vi "AI_Loop.vi"(8 "error in":errorcluster, 10 "AI_Type":T1=enum."TC") -> (0 "error out":errorcluster)   [LabVIEW 2018]
doc: "This example demonstrates how to continuously acquire buffered voltage measurements using a DAQmx device.\n\nFor instructions on how to connect your signals to the DAQ device, refer to your device documentation."
uses:
  Controls/Enums/AI_Type_Enum.ctl
  Controls/Enums/AI_Loop_Enum.ctl
  Controls/Clusts/AI_Loop_Clust.ctl
  Controls/Clusts/AllThresholds.ctl
  Controls/Clusts/ThresholdAlarmLimits.ctl
  Controls/Clusts/Inclinometer_User_Cfg.ctl
  Controls/Clusts/AlarmSettingsClust.ctl
  Controls/Clusts/AlarmThresh_OneChan.ctl
  Controls/Enums/LogLoopEnum.ctl
  Controls/Enums/FP_Loop_Enum.ctl
  Controls/Enums/WatchdogTimer_Enum.ctl
  <vilib>/DAQmx/read.llb/DAQmx Read (Analog 1D DBL NChan 1Samp).vi
  <vilib>/DAQmx/create/channels.llb/DAQmx Create Channel (AI-Voltage-Basic).vi
  <vilib>/DAQmx/create/channels.llb/DAQmx Create Channel (AI-Temperature-Thermocouple).vi
  <vilib>/DAQmx/miscellaneous.llb/DAQmx Fill In Error Info.vi
panel:
  out "Graph":dbl[](graph)
  # "Acquired Data"
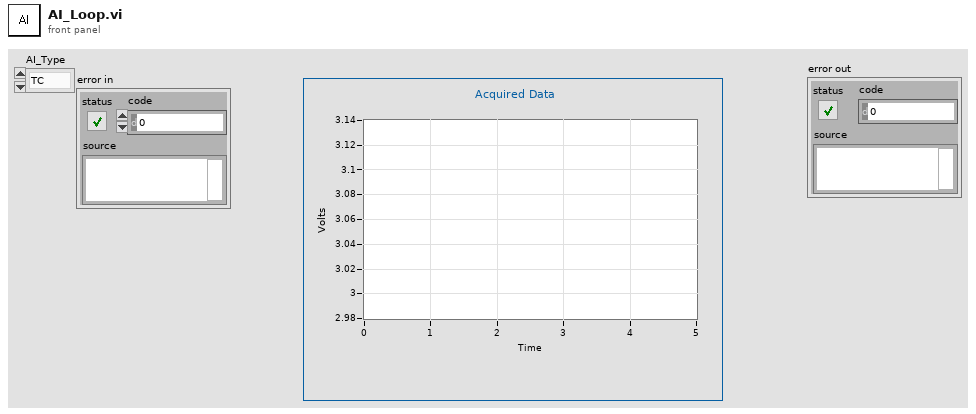
[diagram p1: front panel]
types:
  T1 = typedef "AI_Type_Enum.ctl" = enum16{"AI", "TC"}
  T2 = typedef "AI_Loop_Clust.ctl" = cluster{"AI_Type":T1, "task":refnum<k21>, "AllThresholds_deprecated":T3, "Inclin":T5, "Alarm":T6}
  T3 = typedef "AllThresholds.ctl" = cluster{"TC0":T4, "TC1":T4, "TC2":T4, "TC3":T4, "TC4":T4, "TC5":T4, "TC6":T4, "TC7":T4, "TC8":T4, "TC9":T4, "TC10":T4, "TC11":T4, "TC12":T4, "TC13":T4, "TC14":T4, "TC15":T4, "TC16":T4, "TC17":T4, "TC18":T4, "TC19":T4, "TC20":T4, "AI0":T4, "AI1":T4, "AI2":T4, "AI3":T4, "AI4":T4, "AI5":T4, "AI6":T4, "AI7":T4, "AI16":T4, "AI17":T4, "AI18":T4, "AI19":T4, "AI20":T4, "AI21":T4, "AI22":T4, "AI23":T4}
  T4 = typedef "ThresholdAlarmLimits.ctl" = cluster{"Enable":bool, "LoErr":dbl, "LoWarn":dbl, "HiWarn":dbl, "HiErr":dbl, "RX?":bool}
  T5 = typedef "Inclinometer_User_Cfg.ctl" = cluster{"Vmin":dbl, "Vmax":dbl, "Angle_min":dbl, "Angle_max":dbl, "Offset":dbl, "Pos_Neg":bool}
  T6 = typedef "AlarmSettingsClust.ctl" = cluster{"TC13":T7, "AI1":T7, "AI2":T7, "AI3":T7, "AI4":T7, "AI5":T7, "AI6":T7, "AI18":T7, "AI19":T7, "TE1":T7, "TE2":T7, "TE3":T7, "ADAM1":T7, "ADAM2":T7, "ADAM3":T7, "ADAM4":T7, "72CoBeacFreq":T7, "72CoCalFreq":T7, "84CoBeacFreq":T7, "84CoCalFreq":T7, "72Co_CalTonePwr":T7, "72X_CalTonePwr":T7, "84Co_CalTonePwr":T7, "84X_CalTonePwr":T7}
  T7 = typedef "AlarmThresh_OneChan.ctl" = cluster{"Enbl":bool, "ErrsAndWarns":cluster{dbl, dbl, dbl, dbl}}
  T8 = typedef "AI_Loop_Enum.ctl" = enum16{"AI_Init", "AI_Config", "AI_Alarm", "AI_Read", "AI_ChkTime", "AI_Exit"}
  T9 = typedef "WatchdogTimer_Enum.ctl" = enum16{"ResetAll", "CheckAll", "HW1", "HW2", "Tones", "FP", "Noise", "Log", "TCP", "AI", "TC", "ADAM", "Disdrom", "TE", "Weather"}
  T10 = typedef "FP_Loop_Enum.ctl" = enum16{"FP_Init", "FP_Scale", "FP_Tone", "FP_Noise", "FP_Probes", "FP_PXI", "FP_AI", "FP_TC", "FP_PWR_Hist", "FP_Alarm", "FP_Exit"}
  T11 = typedef "LogLoopEnum.ctl" = enum16{"Log_Init", "Log_Config", "Log_CfgAlarm", "Log_TimeDomain", "Log_Tone", "Log_NoiseTrace", "Log_NoiseSum", "Log_DO", "Log_AI", "Log_TC", "Log_Disdrom", "Log_Weather", "Log_TE", "Log_ADAM", "Log_UPS", "Log_ChkTime", "Log_Alarm", "Log_SSH", "Log_Write", "Log_Exit"}
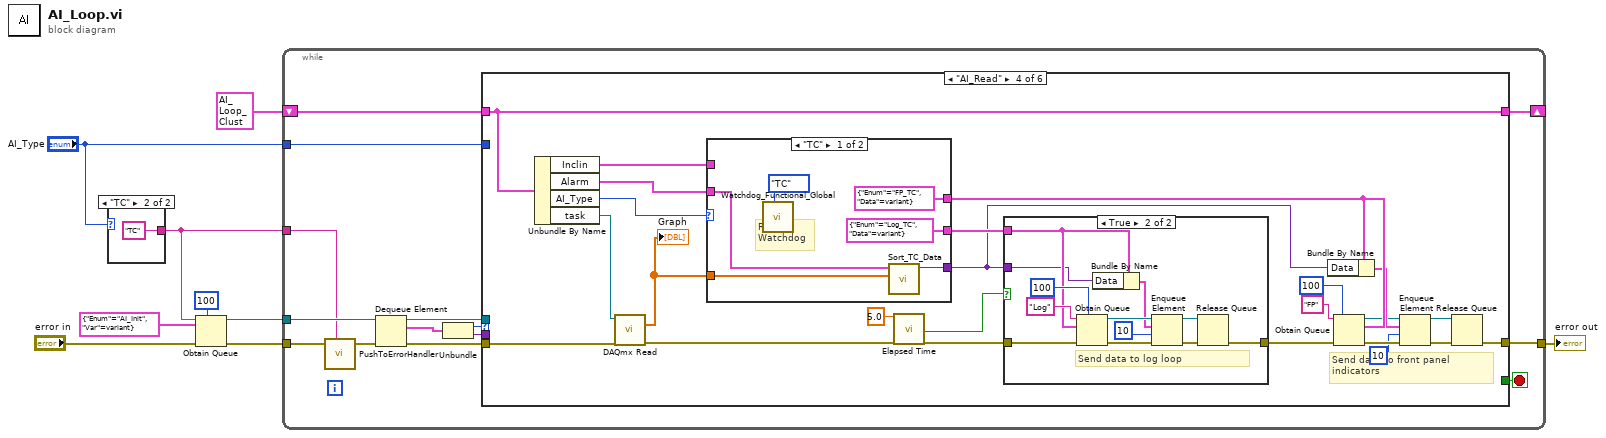
[diagram p0: block diagram]
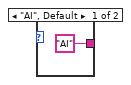
[diagram p2: hidden frame]
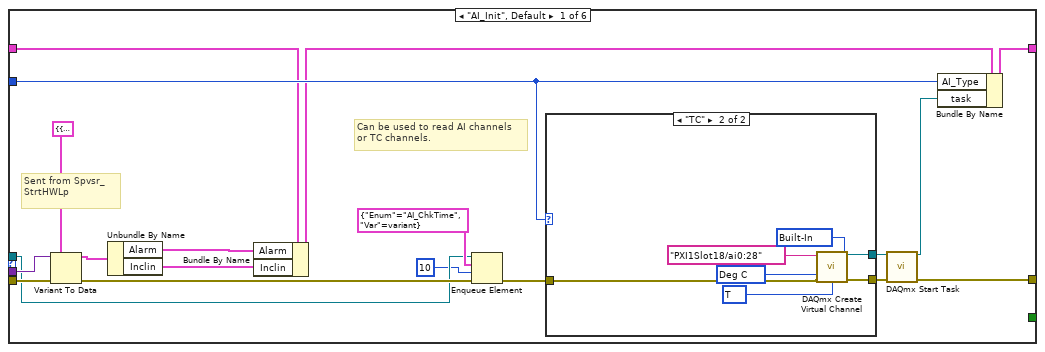
[diagram p3: hidden frame]
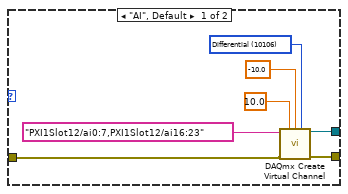
[diagram p4: hidden frame]
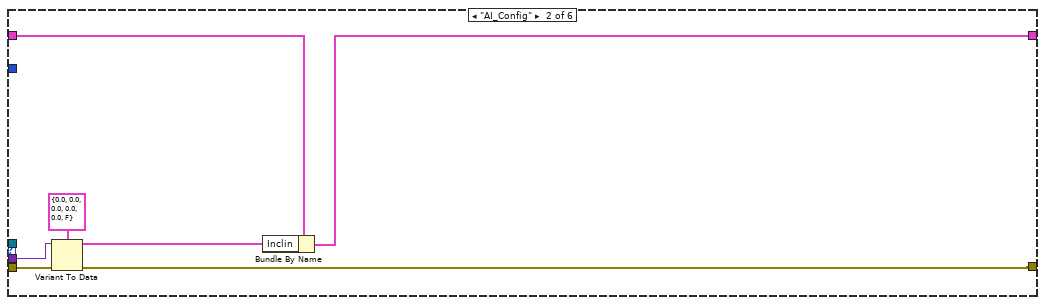
[diagram p5: hidden frame]
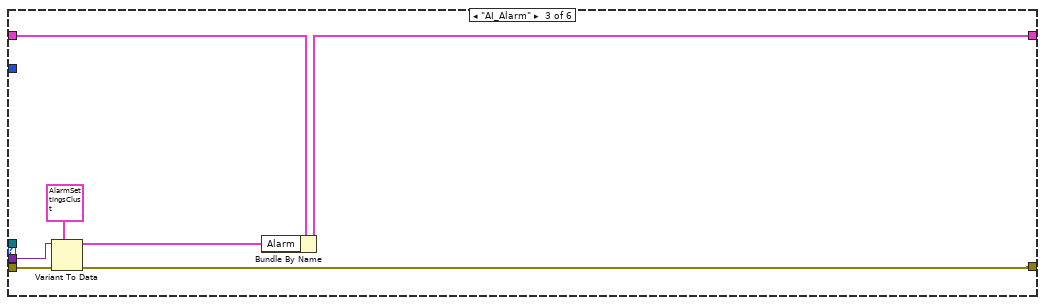
[diagram p6: hidden frame]
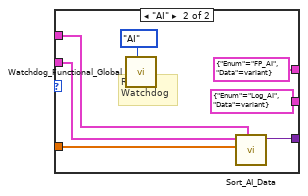
[diagram p8: hidden frame]
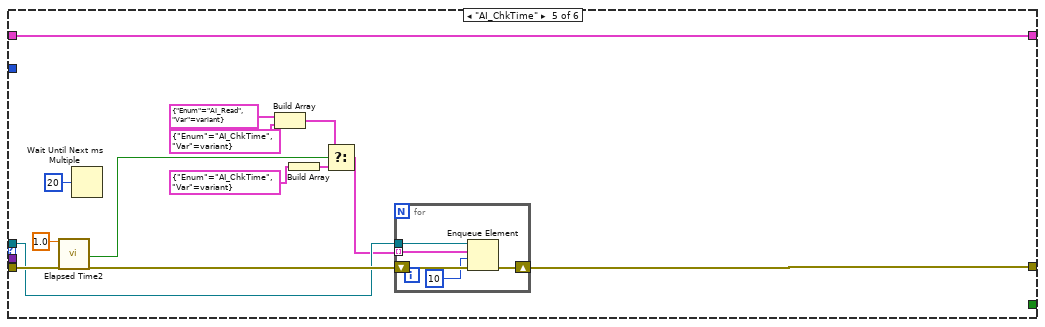
[diagram p9: hidden frame]
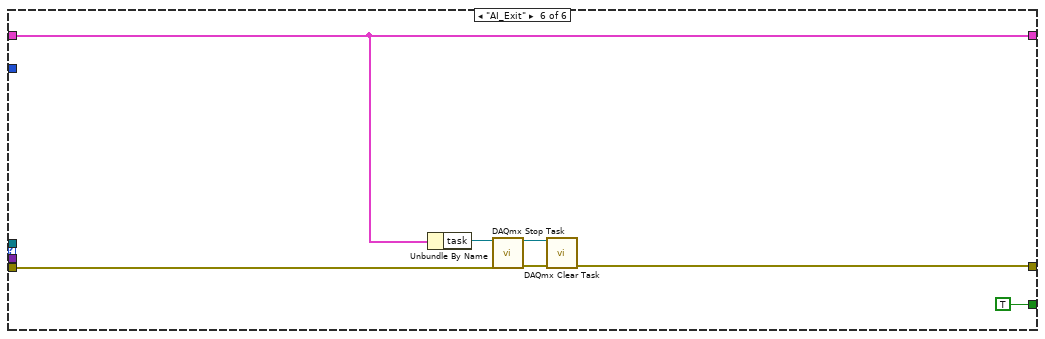
[diagram p10: hidden frame]
diagram:
  n1 = case shown="\"TC\"" "AI_Type" {
    tunnel: ["AI" ("name (unnamed)") "TC" ("name (unnamed)")] -> w4
    frame "AI", Default {
    }
    frame "TC" {
    }
  }
  n2 = Obtain Queue(max queue size (-1, unlimited)=100, name (unnamed)=w4, element data type=cluster{"Enum":T8, "Var":variant} {"Enum"=enum."AI_Init", "Var"=variant}, error in (no error)="error in") -> (queue out=w2:refnum<queue>, error out=w1:errorcluster)  [unwired: 1 in, 1 out]
  n3 = while {
    tunnel: w1 -> [w17]
    tunnel: [w25] -> w6
    tunnel: w2 -> [w19]
    tunnel: w4 -> [w14]
    shift-right: [w12] -> _
    shift-left: T2 {"AI_Type"=enum."TC", "task"="", "AllThresholds_deprecated"={"TC0"={"Enable"=FALSE, "LoErr"=34.0, "LoWarn"=60.0, "HiWarn"=90.0, "HiErr"=105.0, "RX?"=FALSE}, "TC1"={"Enable"=FALSE, "LoErr"=34.0, "LoWarn"=60.0, "HiWarn"=90.0, "HiErr"=105.0, "RX?"=FALSE}, "TC2"={"Enable"=FALSE, "LoErr"=34.0, "LoWarn"=60.0, "HiWarn"=90.0, "HiErr"=105.0, "RX?"=FALSE}, "TC3"={"Enable"=FALSE, "LoErr"=34.0, "LoWarn"=60.0, "HiWarn"=90.0, "HiErr"=105.0, "RX?"=FALSE}, "TC4"={"Enable"=FALSE, "LoErr"=34.0, "LoWarn"=60.0, "HiWarn"=90.0, "HiErr"=105.0, "RX?"=FALSE}, "TC5"={"Enable"=FALSE, "LoErr"=34.0, "LoWarn"=60.0, "HiWarn"=90.0, "HiErr"=105.0, "RX?"=FALSE}, "TC6"={"Enable"=FALSE, "LoErr"=34.0, "LoWarn"=60.0, "HiWarn"=90.0, "HiErr"=105.0, "RX?"=FALSE}, "TC7"={"Enable"=FALSE, "LoErr"=34.0, "LoWarn"=60.0, "HiWarn"=90.0, "HiErr"=105.0, "RX?"=FALSE}, "TC8"={"Enable"=FALSE, "LoErr"=34.0, "LoWarn"=60.0, "HiWarn"=90.0, "HiErr"=105.0, "RX?"=FALSE}, "TC9"={"Enable"=FALSE, "LoErr"=34.0, "LoWarn"=60.0, "HiWarn"=90.0, "HiErr"=105.0, "RX?"=FALSE}, "TC10"={"Enable"=FALSE, "LoErr"=34.0, "LoWarn"=60.0, "HiWarn"=90.0, "HiErr"=105.0, "RX?"=FALSE}, "TC11"={"Enable"=FALSE, "LoErr"=34.0, "LoWarn"=60.0, "HiWarn"=90.0, "HiErr"=105.0, "RX?"=FALSE}, "TC12"={"Enable"=FALSE, "LoErr"=34.0, "LoWarn"=60.0, "HiWarn"=90.0, "HiErr"=105.0, "RX?"=FALSE}, "TC13"={"Enable"=FALSE, "LoErr"=34.0, "LoWarn"=60.0, "HiWarn"=90.0, "HiErr"=105.0, "RX?"=FALSE}, "TC14"={"Enable"=FALSE, "LoErr"=34.0, "LoWarn"=60.0, "HiWarn"=90.0, "HiErr"=105.0, "RX?"=FALSE}, "TC15"={"Enable"=FALSE, "LoErr"=34.0, "LoWarn"=60.0, "HiWarn"=90.0, "HiErr"=105.0, "RX?"=FALSE}, "TC16"={"Enable"=FALSE, "LoErr"=34.0, "LoWarn"=60.0, "HiWarn"=90.0, "HiErr"=105.0, "RX?"=FALSE}, "TC17"={"Enable"=FALSE, "LoErr"=34.0, "LoWarn"=60.0, "HiWarn"=90.0, "HiErr"=105.0, "RX?"=FALSE}, "TC18"={"Enable"=FALSE, "LoErr"=34.0, "LoWarn"=60.0, "HiWarn"=90.0, "HiErr"=105.0, "RX?"=FALSE}, "TC19"={"Enable"=FALSE, "LoErr"=34.0, "LoWarn"=60.0, "HiWarn"=90.0, "HiErr"=105.0, "RX?"=FALSE}, "TC20"={"Enable"=FALSE, "LoErr"=34.0, "LoWarn"=60.0, "HiWarn"=90.0, "HiErr"=105.0, "RX?"=FALSE}, "AI0"={"Enable"=FALSE, "LoErr"=0.0, "LoWarn"=2.0, "HiWarn"=0.0, "HiErr"=0.0, "RX?"=TRUE}, "AI1"={"Enable"=FALSE, "LoErr"=0.0, "LoWarn"=0.0, "HiWarn"=0.0, "HiErr"=0.0, "RX?"=TRUE}, "AI2"={"Enable"=FALSE, "LoErr"=0.0, "LoWarn"=0.0, "HiWarn"=0.0, "HiErr"=0.0, "RX?"=TRUE}, "AI3"={"Enable"=FALSE, "LoErr"=0.0, "LoWarn"=0.0, "HiWarn"=0.0, "HiErr"=0.0, "RX?"=TRUE}, "AI4"={"Enable"=FALSE, "LoErr"=0.0, "LoWarn"=0.0, "HiWarn"=0.0, "HiErr"=0.0, "RX?"=TRUE}, "AI5"={"Enable"=FALSE, "LoErr"=0.0, "LoWarn"=0.0, "HiWarn"=0.0, "HiErr"=0.0, "RX?"=TRUE}, "AI6"={"Enable"=FALSE, "LoErr"=0.0, "LoWarn"=0.0, "HiWarn"=0.0, "HiErr"=0.0, "RX?"=TRUE}, "AI7"={"Enable"=FALSE, "LoErr"=0.0, "LoWarn"=0.0, "HiWarn"=0.0, "HiErr"=0.0, "RX?"=FALSE}, "AI16"={"Enable"=FALSE, "LoErr"=0.0, "LoWarn"=0.0, "HiWarn"=0.0, "HiErr"=0.0, "RX?"=FALSE}, "AI17"={"Enable"=FALSE, "LoErr"=0.0, "LoWarn"=0.0, "HiWarn"=0.0, "HiErr"=0.0, "RX?"=FALSE}, "AI18"={"Enable"=FALSE, "LoErr"=0.0, "LoWarn"=0.0, "HiWarn"=0.0, "HiErr"=0.0, "RX?"=FALSE}, "AI19"={"Enable"=FALSE, "LoErr"=0.0, "LoWarn"=0.0, "HiWarn"=0.0, "HiErr"=0.0, "RX?"=FALSE}, "AI20"={"Enable"=FALSE, "LoErr"=0.0, "LoWarn"=0.0, "HiWarn"=0.0, "HiErr"=0.0, "RX?"=FALSE}, "AI21"={"Enable"=FALSE, "LoErr"=0.0, "LoWarn"=0.0, "HiWarn"=0.0, "HiErr"=0.0, "RX?"=FALSE}, "AI22"={"Enable"=FALSE, "LoErr"=0.0, "LoWarn"=0.0, "HiWarn"=0.0, "HiErr"=0.0, "RX?"=FALSE}, "AI23"={"Enable"=FALSE, "LoErr"=0.0, "LoWarn"=0.0, "HiWarn"=0.0, "HiErr"=0.0, "RX?"=FALSE}}, "Inclin"={"Vmin"=0.0, "Vmax"=0.0, "Angle_min"=0.0, "Angle_max"=0.0, "Offset"=0.0, "Pos_Neg"=FALSE}, "Alarm"={"TC13"={"Enbl"=FALSE, "ErrsAndWarns"={0.0, 0.0, 0.0, 0.0}}, "AI1"={"Enbl"=FALSE, "ErrsAndWarns"={0.0, 0.0, 0.0, 0.0}}, "AI2"={"Enbl"=FALSE, "ErrsAndWarns"={0.0, 0.0, 0.0, 0.0}}, "AI3"={"Enbl"=FALSE, "ErrsAndWarns"={0.0, 0.0, 0.0, 0.0}}, "AI4"={"Enbl"=FALSE, "ErrsAndWarns"={0.0, 0.0, 0.0, 0.0}}, "AI5"={"Enbl"=FALSE, "ErrsAndWarns"={0.0, 0.0, 0.0, 0.0}}, "AI6"={"Enbl"=FALSE, "ErrsAndWarns"={0.0, 0.0, 0.0, 0.0}}, "AI18"={"Enbl"=FALSE, "ErrsAndWarns"={0.0, 0.0, 0.0, 0.0}}, "AI19"={"Enbl"=FALSE, "ErrsAndWarns"={0.0, 0.0, 0.0, 0.0}}, "TE1"={"Enbl"=FALSE, "ErrsAndWarns"={0.0, 0.0, 0.0, 0.0}}, "TE2"={"Enbl"=FALSE, "ErrsAndWarns"={0.0, 0.0, 0.0, 0.0}}, "TE3"={"Enbl"=FALSE, "ErrsAndWarns"={0.0, 0.0, 0.0, 0.0}}, "ADAM1"={"Enbl"=FALSE, "ErrsAndWarns"={0.0, 0.0, 0.0, 0.0}}, "ADAM2"={"Enbl"=FALSE, "ErrsAndWarns"={0.0, 0.0, 0.0, 0.0}}, "ADAM3"={"Enbl"=FALSE, "ErrsAndWarns"={0.0, 0.0, 0.0, 0.0}}, "ADAM4"={"Enbl"=FALSE, "ErrsAndWarns"={0.0, 0.0, 0.0, 0.0}}, "72CoBeacFreq"={"Enbl"=FALSE, "ErrsAndWarns"={0.0, 0.0, 0.0, 0.0}}, "72CoCalFreq"={"Enbl"=FALSE, "ErrsAndWarns"={0.0, 0.0, 0.0, 0.0}}, "84CoBeacFreq"={"Enbl"=FALSE, "ErrsAndWarns"={0.0, 0.0, 0.0, 0.0}}, "84CoCalFreq"={"Enbl"=FALSE, "ErrsAndWarns"={0.0, 0.0, 0.0, 0.0}}, "72Co_CalTonePwr"={"Enbl"=FALSE, "ErrsAndWarns"={0.0, 0.0, 0.0, 0.0}}, "72X_CalTonePwr"={"Enbl"=FALSE, "ErrsAndWarns"={0.0, 0.0, 0.0, 0.0}}, "84Co_CalTonePwr"={"Enbl"=FALSE, "ErrsAndWarns"={0.0, 0.0, 0.0, 0.0}}, "84X_CalTonePwr"={"Enbl"=FALSE, "ErrsAndWarns"={0.0, 0.0, 0.0, 0.0}}}} -> [w13]
    tunnel: "AI_Type" -> [w15]
    stop <- w24 stop-if-true
    n4 = call "PushToErrorHandler.vi"("ErrorIn"=w17, "ErrorLocation"=w14) -> ("ErrorOut"=w16:errorcluster)  [unwired: 5 in]
    n5 = Dequeue Element(queue=w19, error in (no error)=w16) -> (queue out=w18:refnum<queue>, element=w22:cluster{"Enum":T8, "Var":variant}, error out=w23:errorcluster)  [unwired: 1 in, 1 out]
    n6 = Unbundle(w22) -> ("Enum"=w21:T8, "Var"=w20:variant)
    n7 = case shown="\"AI_Read\"" w21 {
      tunnel: [w42 w59 w67 w80 w136 w145] -> w25
      tunnel: [_ _ _ _ _ TRUE ("Stop")] -> w24
      tunnel: w23 -> [w36 w65 w72 w96 w135 w146]
      tunnel: w20 -> [w34 w61 w69 _ _ _]
      tunnel: w18 -> [w33 _ _ _ w131 _]
      tunnel: w15 -> [w39 _ _ _ _ _]
      tunnel: w13 -> [w32 w63 w70 w87 w123 w143]
      tunnel: [w37 w64 w71 w87 w123 w143] -> w12
      frame "AI_Init", Default {
        # "Sent from Spvsr_StrtHWLp"
        # "Can be used to read AI channels\nor TC channels."
        n8 = Variant To Data(error in=w36, type=cluster{"Alarm":T6, "Inclin":T5} {"Alarm"={"TC13"={"Enbl"=FALSE, "ErrsAndWarns"={0.0, 0.0, 0.0, 0.0}}, "AI1"={"Enbl"=FALSE, "ErrsAndWarns"={0.0, 0.0, 0.0, 0.0}}, "AI2"={"Enbl"=FALSE, "ErrsAndWarns"={0.0, 0.0, 0.0, 0.0}}, "AI3"={"Enbl"=FALSE, "ErrsAndWarns"={0.0, 0.0, 0.0, 0.0}}, "AI4"={"Enbl"=FALSE, "ErrsAndWarns"={0.0, 0.0, 0.0, 0.0}}, "AI5"={"Enbl"=FALSE, "ErrsAndWarns"={0.0, 0.0, 0.0, 0.0}}, "AI6"={"Enbl"=FALSE, "ErrsAndWarns"={0.0, 0.0, 0.0, 0.0}}, "AI18"={"Enbl"=FALSE, "ErrsAndWarns"={0.0, 0.0, 0.0, 0.0}}, "AI19"={"Enbl"=FALSE, "ErrsAndWarns"={0.0, 0.0, 0.0, 0.0}}, "TE1"={"Enbl"=FALSE, "ErrsAndWarns"={0.0, 0.0, 0.0, 0.0}}, "TE2"={"Enbl"=FALSE, "ErrsAndWarns"={0.0, 0.0, 0.0, 0.0}}, "TE3"={"Enbl"=FALSE, "ErrsAndWarns"={0.0, 0.0, 0.0, 0.0}}, "ADAM1"={"Enbl"=FALSE, "ErrsAndWarns"={0.0, 0.0, 0.0, 0.0}}, "ADAM2"={"Enbl"=FALSE, "ErrsAndWarns"={0.0, 0.0, 0.0, 0.0}}, "ADAM3"={"Enbl"=FALSE, "ErrsAndWarns"={0.0, 0.0, 0.0, 0.0}}, "ADAM4"={"Enbl"=FALSE, "ErrsAndWarns"={0.0, 0.0, 0.0, 0.0}}, "72CoBeacFreq"={"Enbl"=FALSE, "ErrsAndWarns"={0.0, 0.0, 0.0, 0.0}}, "72CoCalFreq"={"Enbl"=FALSE, "ErrsAndWarns"={0.0, 0.0, 0.0, 0.0}}, "84CoBeacFreq"={"Enbl"=FALSE, "ErrsAndWarns"={0.0, 0.0, 0.0, 0.0}}, "84CoCalFreq"={"Enbl"=FALSE, "ErrsAndWarns"={0.0, 0.0, 0.0, 0.0}}, "72Co_CalTonePwr"={"Enbl"=FALSE, "ErrsAndWarns"={0.0, 0.0, 0.0, 0.0}}, "72X_CalTonePwr"={"Enbl"=FALSE, "ErrsAndWarns"={0.0, 0.0, 0.0, 0.0}}, "84Co_CalTonePwr"={"Enbl"=FALSE, "ErrsAndWarns"={0.0, 0.0, 0.0, 0.0}}, "84X_CalTonePwr"={"Enbl"=FALSE, "ErrsAndWarns"={0.0, 0.0, 0.0, 0.0}}}, "Inclin"={"Vmin"=0.0, "Vmax"=0.0, "Angle_min"=0.0, "Angle_max"=0.0, "Offset"=0.0, "Pos_Neg"=FALSE}} ("cluster"), Variant=w34) -> (data=w30:cluster{"Alarm":T6, "Inclin":T5}, error out=w35:errorcluster)
        n9 = Unbundle By Name(w30) -> ("Alarm"=w27:T6, "Inclin"=w29:T5)
        n10 = Bundle By Name(cluster=w32, "Alarm"=w27, "Inclin"=w29) -> (w31:T2)
        n11 = Enqueue Element(queue=w33, element=cluster{"Enum":T8, "Var":variant} {"Enum"=enum."AI_ChkTime", "Var"=variant}, timeout in ms (-1)=10, error in (no error)=w35) -> (error out=w41:errorcluster)  [unwired: 2 out]
        n12 = case shown="\"TC\"" w39 {
          tunnel: [w48 w57] -> w44
          tunnel: [w47 w56] -> w43
          tunnel: w41 -> [w46 w55]
          frame "AI", Default {
            w49 = 10106 items=["default"=-1, "RSE"=10083, "NRSE"=10078, "Differential"=10106, "Pseudodifferential"=12529] ("Terminal Configuration")
            n13 = call-poly <vilib>:"DAQmx Create Virtual Channel.vi"("maximum value"=10.0 ("Max Voltage"), "minimum value"=-10.0 ("Min Voltage"), "input terminal configuration"=w49, "physical channels"=tag "PXI1Slot12/ai0:7,PXI1Slot12/ai16:23" ("Physical Channel"), "error in"=w46) -> ("task out"=w48:refnum<k21>, "error out"=w47:errorcluster)  [unwired: 9 in]
          }
          frame "TC" {
            w52 = 10086 items=["J"=10072, "K"=10073, "N"=10077, "R"=10082, "S"=10085, "T"=10086, "B"=10047, "E"=10055] ("thermocouple type")
            w53 = 10200 items=["Built-In"=10200, "Constant Value"=10116, "Channel"=10113] ("cjc source")
            w54 = 10143 items=["Deg C"=10143, "Deg F"=10144, "Kelvins"=10325, "Deg R"=10145, "From Custom Scale"=10065] ("units")
            n14 = call-poly <vilib>:"DAQmx Create Virtual Channel.vi"("physical channels"=tag "PXI1Slot18/ai0:28" ("Physical Channel"), "cjc source"=w53, "units"=w54, "error in"=w55, "thermocouple type"=w52) -> ("task out"=w57:refnum<k21>, "error out"=w56:errorcluster)  [unwired: 9 in]
          }
        }
        n15 = call <vilib>:"DAQmx Start Task.vi"("task/channels in"=w44, "error in"=w43) -> ("task out"=w38:refnum<k21>, "error out"=w42:errorcluster)  [unwired: 12 in]
        n16 = Bundle By Name(cluster=w31, "AI_Type"=w39, "task"=w38) -> (w37:T2)
      }
      frame "AI_Config" {
        n17 = Variant To Data(error in=w65, type=T5 {"Vmin"=0.0, "Vmax"=0.0, "Angle_min"=0.0, "Angle_max"=0.0, "Offset"=0.0, "Pos_Neg"=FALSE} ("Inclin"), Variant=w61) -> (data=w60:T5, error out=w59:errorcluster)
        n18 = Bundle By Name(cluster=w63, "Inclin"=w60) -> (w64:T2)
      }
      frame "AI_Alarm" {
        n19 = Variant To Data(error in=w72, type=T6 {"TC13"={"Enbl"=FALSE, "ErrsAndWarns"={0.0, 5.663716814159292, 7.168141592920354, 8.584070796460177}}, "AI1"={"Enbl"=FALSE, "ErrsAndWarns"={0.0, 5.663716814159292, 7.168141592920354, 8.584070796460177}}, "AI2"={"Enbl"=FALSE, "ErrsAndWarns"={0.0, 5.663716814159292, 7.168141592920354, 8.584070796460177}}, "AI3"={"Enbl"=FALSE, "ErrsAndWarns"={0.0, 5.663716814159292, 7.168141592920354, 8.584070796460177}}, "AI4"={"Enbl"=FALSE, "ErrsAndWarns"={0.0, 5.663716814159292, 7.168141592920354, 8.584070796460177}}, "AI5"={"Enbl"=FALSE, "ErrsAndWarns"={0.0, 5.663716814159292, 7.168141592920354, 8.584070796460177}}, "AI6"={"Enbl"=FALSE, "ErrsAndWarns"={0.0, 5.663716814159292, 7.168141592920354, 8.584070796460177}}, "AI18"={"Enbl"=FALSE, "ErrsAndWarns"={0.0, 5.663716814159292, 7.168141592920354, 8.584070796460177}}, "AI19"={"Enbl"=FALSE, "ErrsAndWarns"={0.0, 5.663716814159292, 7.168141592920354, 8.584070796460177}}, "TE1"={"Enbl"=FALSE, "ErrsAndWarns"={0.0, 5.663716814159292, 7.168141592920354, 8.584070796460177}}, "TE2"={"Enbl"=FALSE, "ErrsAndWarns"={0.0, 5.663716814159292, 7.168141592920354, 8.584070796460177}}, "TE3"={"Enbl"=FALSE, "ErrsAndWarns"={0.0, 5.663716814159292, 7.168141592920354, 8.584070796460177}}, "ADAM1"={"Enbl"=FALSE, "ErrsAndWarns"={0.0, 5.663716814159292, 7.168141592920354, 8.584070796460177}}, "ADAM2"={"Enbl"=FALSE, "ErrsAndWarns"={0.0, 5.663716814159292, 7.168141592920354, 8.584070796460177}}, "ADAM3"={"Enbl"=FALSE, "ErrsAndWarns"={0.0, 5.663716814159292, 7.168141592920354, 8.584070796460177}}, "ADAM4"={"Enbl"=FALSE, "ErrsAndWarns"={0.0, 5.663716814159292, 7.168141592920354, 8.584070796460177}}, "72CoBeacFreq"={"Enbl"=FALSE, "ErrsAndWarns"={0.0, 5.663716814159292, 7.168141592920354, 8.584070796460177}}, "72CoCalFreq"={"Enbl"=FALSE, "ErrsAndWarns"={0.0, 5.663716814159292, 7.168141592920354, 8.584070796460177}}, "84CoBeacFreq"={"Enbl"=FALSE, "ErrsAndWarns"={0.0, 5.663716814159292, 7.168141592920354, 8.584070796460177}}, "84CoCalFreq"={"Enbl"=FALSE, "ErrsAndWarns"={0.0, 5.663716814159292, 7.168141592920354, 8.584070796460177}}, "72Co_CalTonePwr"={"Enbl"=FALSE, "ErrsAndWarns"={0.0, 5.663716814159292, 7.168141592920354, 8.584070796460177}}, "72X_CalTonePwr"={"Enbl"=FALSE, "ErrsAndWarns"={0.0, 5.663716814159292, 7.168141592920354, 8.584070796460177}}, "84Co_CalTonePwr"={"Enbl"=FALSE, "ErrsAndWarns"={0.0, 5.663716814159292, 7.168141592920354, 8.584070796460177}}, "84X_CalTonePwr"={"Enbl"=FALSE, "ErrsAndWarns"={0.0, 5.663716814159292, 7.168141592920354, 8.584070796460177}}} ("Alarm"), Variant=w69) -> (data=w68:T6, error out=w67:errorcluster)
        n20 = Bundle By Name(cluster=w70, "Alarm"=w68) -> (w71:T2)
      }
      frame "AI_Read" {
        # "Send data to front panel\nindicators"
        n21 = Unbundle By Name(w87) -> ("Inclin"=w74:T5, "Alarm"=w84:T6, "AI_Type"=w86:T1, "task"=w85:refnum<k21>)
        n22 = call-poly <vilib>:"DAQmx Read.vi"("task/channels in"=w85, "error in"=w96) -> ("data"=w94:dbl[], "error out"=w79:errorcluster)  [unwired: 11 in, 1 out]
        "Graph" <- w94
        n23 = case shown="\"TC\"" w86 {
          tunnel: [cluster{"Enum":T11, "Data":variant} {"Enum"=enum."Log_TC", "Data"=variant} cluster{"Enum":T11, "Data":variant} {"Enum"=enum."Log_AI", "Data"=variant}] -> w95
          tunnel: w94 -> [w112 w119]
          tunnel: [w114 w121] -> w75
          tunnel: [cluster{"Enum":T10, "Data":variant} {"Enum"=enum."FP_TC", "Data"=variant} cluster{"Enum":T10, "Data":variant} {"Enum"=enum."FP_AI", "Data"=variant}] -> w90
          tunnel: w84 -> [w111 w118]
          tunnel: w74 -> [_ w117]
          frame "TC" {
            # "Reset\nWatchdog"
            n24 = call "Watchdog_Functional_Global.vi"("Watchdog"=WatchdogTimer_Enum."TC") -> ()  [unwired: 10 in, 1 out]
            n25 = call "Sort_TC_Data.vi"("TC_data"=w112, "AlarmSettings"=w111) -> ("TC_Variant"=w114:variant)  [unwired: 9 in]
          }
          frame "AI" {
            # "Reset\nWatchdog"
            n26 = call "Watchdog_Functional_Global.vi"("Watchdog"=WatchdogTimer_Enum."AI") -> ()  [unwired: 10 in, 1 out]
            n27 = call "Sort_AI_Data.vi"("Inclin"=w117, "AI_data"=w119, "AlarmSettings"=w118) -> ("AI_Variant"=w121:variant)  [unwired: 7 in, 1 out]
          }
        }
        n28 = call "Elapsed Time"("Time Target (s)"=5.0, "error in (no error)"=w79) -> ("Time has Elapsed"=w77:bool, "error out"=w78:errorcluster)  [unwired: 10 in, 6 out]
        n29 = case shown="True" w77 {
          tunnel: w78 -> [w97 w105]
          tunnel: w95 -> [_ w103]
          tunnel: w75 -> [_ w102]
          tunnel: [w97 w99] -> w83
          frame False {
          }
          frame True {
            # "Send data to log loop"
            n30 = Obtain Queue(max queue size (-1, unlimited)=100, name (unnamed)="Log", element data type=w103, error in (no error)=w105) -> (queue out=w107:refnum<queue>, error out=w106:errorcluster)  [unwired: 1 in, 1 out]
            n31 = Bundle By Name(cluster=w103, "Data"=w102) -> (w104:cluster{"Enum":T11, "Data":variant})
            n32 = Enqueue Element(queue=w107, element=w104, timeout in ms (-1)=10, error in (no error)=w106) -> (queue out=w101:refnum<queue>, error out=w100:errorcluster)  [unwired: 1 out]
            n33 = Release Queue(queue=w101, error in (no error)=w100) -> (error out=w99:errorcluster)  [unwired: 1 in, 2 out]
          }
        }
        n34 = Bundle By Name(cluster=w90, "Data"=w75) -> (w89:cluster{"Enum":T10, "Data":variant})
        n35 = Obtain Queue(max queue size (-1, unlimited)=100, name (unnamed)="FP", element data type=w90, error in (no error)=w83) -> (queue out=w88:refnum<queue>, error out=w91:errorcluster)  [unwired: 1 in, 1 out]
        n36 = Enqueue Element(queue=w88, element=w89, timeout in ms (-1)=10, error in (no error)=w91) -> (queue out=w82:refnum<queue>, error out=w81:errorcluster)  [unwired: 1 out]
        n37 = Release Queue(queue=w82, error in (no error)=w81) -> (error out=w80:errorcluster)  [unwired: 1 in, 2 out]
      }
      frame "AI_ChkTime" {
        n38 = call "Elapsed Time2"("Time Target (s)"=1.0, "error in (no error)"=w135) -> ("Time has Elapsed"=w129:bool, "error out"=w134:errorcluster)  [unwired: 10 in, 6 out]
        n39 = Wait Until Next ms Multiple(millisecond multiple=u32 20 ("milliseconds to wait")) -> ()  [unwired: 1 out]
        n40 = Build Array(cluster{"Enum":T8, "Var":variant} {"Enum"=enum."AI_Read", "Var"=variant} ("element"), cluster{"Enum":T8, "Var":variant} {"Enum"=enum."AI_ChkTime", "Var"=variant} ("element")) -> (w127:cluster{"Enum":T8, "Var":variant}[])
        n41 = Build Array(cluster{"Enum":T8, "Var":variant} {"Enum"=enum."AI_ChkTime", "Var"=variant} ("element")) -> (w124:cluster{"Enum":T8, "Var":variant}[])
        n42 = Select(t=w127, s=w129, f=w124) -> (s? t:f=w130:cluster{"Enum":T8, "Var":variant}[])
        n43 = for {
          tunnel: w131 -> [w139]
          tunnel: w130 -> [w138] mode=indexing
          shift-right: [w141] -> w136
          shift-left: w134 -> [w140]
          n44 = Enqueue Element(queue=w139, element=w138, timeout in ms (-1)=10, error in (no error)=w140) -> (error out=w141:errorcluster)  [unwired: 2 out]
        }
      }
      frame "AI_Exit" {
        n45 = Unbundle By Name(w143) -> ("task"=w142:refnum<k21>)
        n46 = call <vilib>:"DAQmx Stop Task.vi"("task/channels in"=w142, "error in"=w146) -> ("task out"=w148:refnum<k21>, "error out"=w147:errorcluster)  [unwired: 12 in]
        n47 = call <vilib>:"DAQmx Clear Task.vi"("task in"=w148, "error in"=w147) -> ("error out"=w145:errorcluster)  [unwired: 13 in]
      }
    }
  }
  "error out" <- w6
